vi "Arm Control.vi"(10 "Starting Arm Value":dbl, 11 "Input":dbl) -> (2 "Arm Angle":dbl, 3 "Shooter Speed":dbl)   [LabVIEW 2015]
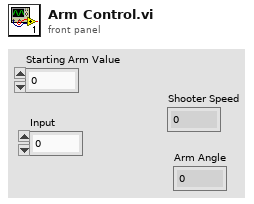
[diagram p1: front panel]
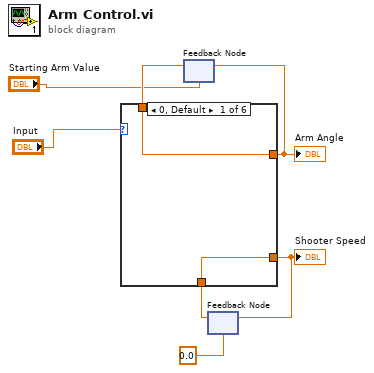
[diagram p0: block diagram]
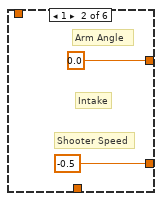
[diagram p2: hidden frame]
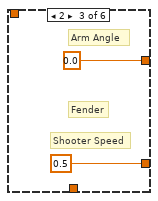
[diagram p3: hidden frame]
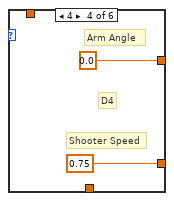
[diagram p4: hidden frame]
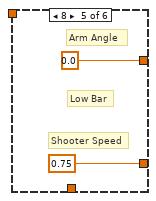
[diagram p5: hidden frame]
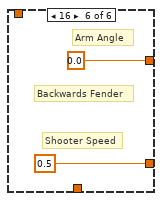
[diagram p6: hidden frame]
diagram:
  n1 = feedback #1("Starting Arm Value") -> (w2:dbl)
  n2 = feedback #2(0.0) -> (w5:dbl)
  n3 = case shown="0, Default" "Input" {
    tunnel: [w9 -0.5 0.5 0.75 0.75 0.5] -> w6
    tunnel: [w8 0.0 0.0 0.0 0.0 0.0] -> w3
    tunnel: w5 -> [w9 _ _ _ _ _]
    tunnel: w2 -> [w8 _ _ _ _ _]
    frame 0, Default {
    }
    frame 1 {
      # "Intake"
      # "Arm Angle"
      # "Shooter Speed"
    }
    frame 2 {
      # "Fender"
      # "Arm Angle"
      # "Shooter Speed"
    }
    frame 4 {
      # "D4"
      # "Arm Angle"
      # "Shooter Speed"
    }
    frame 8 {
      # "Low Bar"
      # "Arm Angle"
      # "Shooter Speed"
    }
    frame 16 {
      # "Backwards Fender"
      # "Arm Angle"
      # "Shooter Speed"
    }
  }
  "Shooter Speed" <- w6
  "Arm Angle" <- w3
  n4 = feedback-in #1(w3) -> ()
  n5 = feedback-in #2(w6) -> ()
